vi "力觉选择计算C.vi"(8 "取绝对值?F":bool, 9 "Pr":T1={"选择"=enum."Fx", "系数x"=1.0, "系数+"=1.0, "上限"=4.3, "下限"=3.7, "Ymax"=50.0, "Ymin"=-50.0, "点数"=1000.0, "锁系数x"=1.0, "锁上限"=0.4, "锁下限"=0.6, "锁系数+"=1.0, "起点"=0.20000000298023224, "终点"=0.6499999761581421, "锁起点"=0.05000000074505806, "锁终点"=0.20000000298023224, "上参考"=4.3, "下参考"=3.7, "基准"=3.7} {"系数+" format="%.3f"; "基准" format="%.2f"; "下参考" format="%.2f"; "上参考" format="%.2f"; "锁终点" format="%.2f"; "锁起点" format="%.2f"; "终点" format="%.2f"; "起点" format="%.2f"; "锁系数+" format="%.3f"; "锁下限" format="%.2f"; "锁上限" format="%.2f"; "锁系数x" format="%.3f"; "下限" format="%.2f"; "上限" format="%.2f"; "系数x" format="%.3f"}, 11 "力":sgl[](array[numeric]) format="%.2f") -> (0 "六曲线":T2, 3 "曲线":sgl)   [LabVIEW 2018]
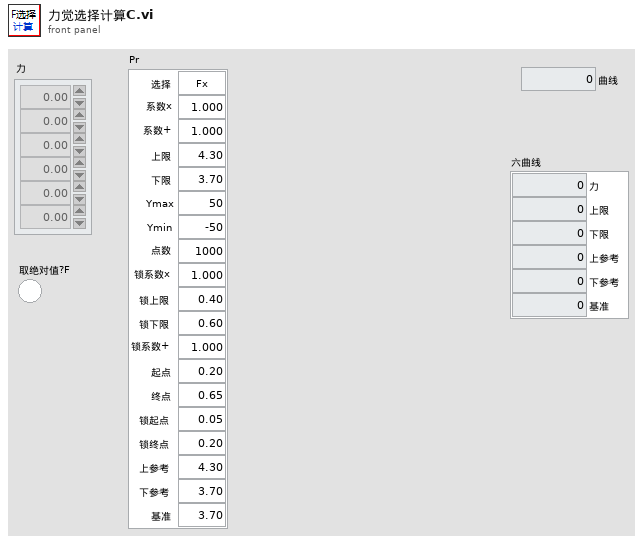
[diagram p1: front panel]
types:
  T1 = cluster{"选择":enum16{"Fx", "Fy", "Fz", "Mx", "My", "Mz"}, "系数x":sgl, "系数+":sgl, "上限":sgl, "下限":sgl, "Ymax":dbl, "Ymin":dbl, "点数":dbl, "锁系数x":sgl, "锁上限":sgl, "锁下限":sgl, "锁系数+":sgl, "起点":dbl, "终点":dbl, "锁起点":dbl, "锁终点":dbl, "上参考":sgl, "下参考":sgl, "基准":sgl}
  T2 = cluster{"力":sgl, "上限":sgl, "下限":sgl, "上参考":sgl, "下参考":sgl, "基准":sgl}
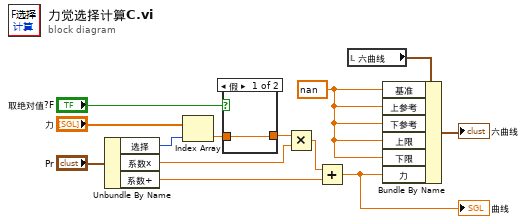
[diagram p0: block diagram]
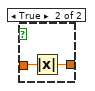
[diagram p2: hidden frame]
diagram:
  w8 = sgl nan
  n1 = Unbundle By Name("Pr") -> ("选择"=w12:enum16{"Fx", "Fy", "Fz", "Mx", "My", "Mz"}, "系数x"=w11:sgl, "系数+"=w3:sgl)
  n2 = Index Array(array="力", index=w12) -> (element=w6:sgl)
  n3 = case shown="假" "取绝对值?F" {
    tunnel: w6 -> [w14 w16]
    tunnel: [w14 w15] -> w5
    frame False {
    }
    frame True {
      n4 = Absolute Value(x=w16) -> (abs(x)=w15:sgl)
    }
  }
  n5 = Multiply(x=w5, y=w11) -> (x*y=w2:sgl)
  n6 = Add(x=w2, y=w3) -> (x+y=w1:sgl)
  "曲线" <- w1
  n7 = local read "六曲线"() -> (w10:T2)
  n8 = Bundle By Name(cluster=w10, "基准"=w8, "上参考"=w8, "下参考"=w8, "上限"=w8, "下限"=w8, "力"=w1) -> (→"六曲线":T2)
